vi "ROS_Master_setMasterPort.vi"(2 "Port":u32=11311, 3 "Wait for real address?":bool, 4 "ROS_Master in":T1) -> (1 "ROS_Master out":T1)   [LabVIEW 2015]
doc: "Sets master port and checks for a valid connection"
uses:
  ROS_Master.ctl
  ROS_Topic.ctl
  ROS_Node.ctl
  ROS_Service.ctl
panel:
  out "Good?":bool
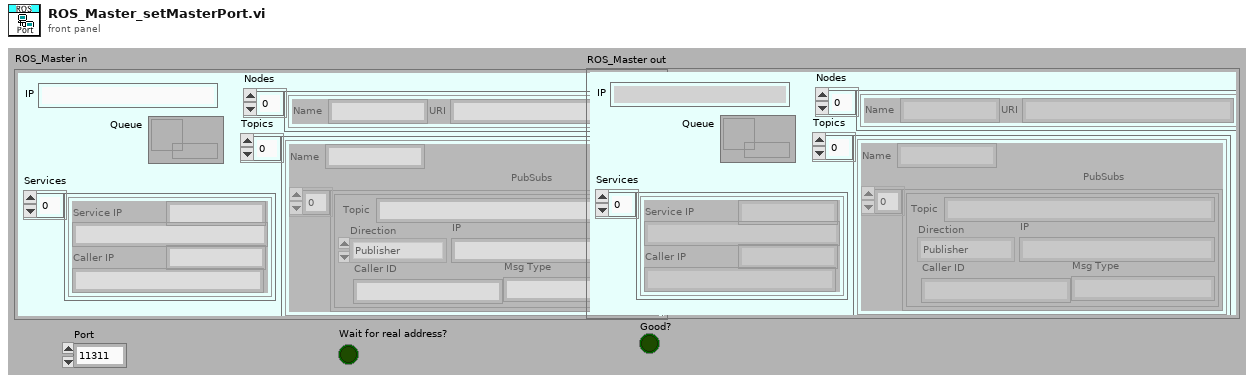
[diagram p1: front panel]
types:
  T1 = typedef "ROS_Master.ctl" = cluster{"IP":string, "Topics":cluster{"Name":string, "PubSubs":T2[]}[], "Nodes":T3[], "Services":T4[], "Queue":refnum<queue>}
  T2 = typedef "ROS_Topic.ctl" = cluster{"Caller ID":string, "IP":string, "Msg Type":string, "Direction":enum16{"Publisher", "Subscriber"}, "Topic":string}
  T3 = typedef "ROS_Node.ctl" = cluster{"Name":string, "URI":string}
  T4 = typedef "ROS_Service.ctl" = cluster{"Service":string, "Service IP":string, "Caller IP":string, "Caller ID":string}
  T5 = enum16{"http://IP:port", "http://IP", "IP:port", "IP only"}
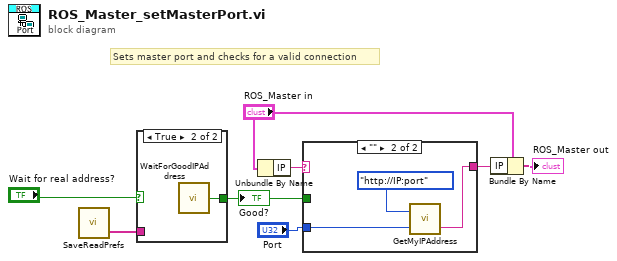
[diagram p0: block diagram]
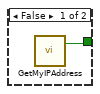
[diagram p2: hidden frame]
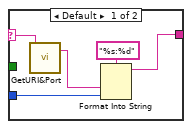
[diagram p3: hidden frame]
diagram:
  # "Sets master port and checks for a valid connection"
  n1 = call "SaveReadPrefs.vi"() -> ("Masters"=w1:string[])  [unwired: 3 in]
  n2 = case shown="True" "Wait for real address?" {
    tunnel: [w9 w10] -> w2
    tunnel: w1 -> [_ _]
    frame False {
      n3 = call "GetMyIPAddress.vi"() -> ("Good?"=w9:bool)  [unwired: 2 in, 1 out]
    }
    frame True {
      n4 = call "WaitForGoodIPAddress.vi"() -> ("Good?"=w10:bool)  [unwired: 1 in]
    }
  }
  "Good?" <- w2
  n5 = Unbundle By Name("ROS_Master in") -> ("IP"=w8:string)
  n6 = case shown="\"\"" w8 {
    selector: w8 -> [w12 _]
    tunnel: [w13 w17] -> w7
    tunnel: "Port" -> [w14 w18]
    tunnel: w2 -> [_ _]
    frame Default {
      n7 = call "GetURI&Port.vi"("URI in"=w12) -> ("URI"=w11:string)  [unwired: 1 out]
      n8 = Format Into String(format string="%s:%d", w11, w14) -> (resulting string=w13:string)  [unwired: 2 in, 1 out]
    }
    frame "" {
      n9 = call "GetMyIPAddress.vi"("Port"=w18, "Format"=T5."http://IP:port") -> ("URI"=w17:string)  [unwired: 1 out]
    }
  }
  n10 = Bundle By Name(cluster="ROS_Master in", "IP"=w7) -> (→"ROS_Master out":T1)
